vi "pressure system controller v18 numatics automated injection.vi"() -> ()   [LabVIEW 2015]
uses:
  <vilib>/DAQmx/write.llb/DAQmx Write (Digital 1D Bool 1Chan 1Samp).vi
  <vilib>/DAQmx/write.llb/DAQmx Write (Analog DBL 1Chan 1Samp).vi
  <vilib>/DAQmx/read.llb/DAQmx Read (Analog DBL 1Chan 1Samp).vi
  <vilib>/DAQmx/create/channels.llb/DAQmx Create Channel (AI-Voltage-Basic).vi
  <vilib>/DAQmx/configure/timing.llb/DAQmx Timing (Sample Clock).vi
  <vilib>/DAQmx/miscellaneous.llb/DAQmx Fill In Error Info.vi
  <vilib>/DAQmx/create/channels.llb/DAQmx Create Channel (AO-Voltage-Basic).vi
  <vilib>/DAQmx/create/channels.llb/DAQmx Create Channel (DO-Digital Output).vi
  <vilib>/express/express shared/transition.llb/Dynamic To Waveform Array.vi
  <vilib>/express/express signal manip/GetorSetDDTAttributes/Set DDT Attributes/SetT0.vi
  <vilib>/express/express shared/transition.llb/Waveform Array To Dynamic.vi
  <instrlib>/Keithley 24XX/Public/Data/Read (Single Point).vi
  <vilib>/express/express signal manip/GetorSetDDTAttributes/Set DDT Attributes/Set DDT Properties.xnode
  <vilib>/ptbypt/NI_PtbyPt.lvlib
  <instrlib>/Keithley 24XX/Keithley 24XX.lvlib
  <instrlib>/Agilent E4980/Agilent E4980.lvlib
panel:
  out "auto loop stop":bool
  in  "MUX1: LCR (+) 2":T1(radio)
  in  "Time Delay before current injection (s)":i32=5
  out "Inject Current":bool
  in  "Time Interval (sec)":i32=600
  in  "number of current inject":i32=5
  in  "Turn on (MAKE SURE TURN OFF)":bool=TRUE
  in  "MUX1: LCR (+)":T1(radio)
  in  "MUX2: LCR (-)":T1(radio)
  in  "MUX3: Keithley (+)":T1(radio)
  in  "MUX4: Keithley (-)":T1(radio)
  in  "Write to file":bool=TRUE caption="Enable"
  out "Pressure":dbl
  out "Impedance":dbl format="%^#_6e"
  out "Phase (deg)":dbl
  in  "Function (0: Cp-D)":u16(ring)=17 items=["Cp-D", "Cp-Q", "Cp-G", "Cp-Rp", "Cs-D", "Cs-Q", "Cs-Rs", "Lp-D", "Lp-Q", "Lp-G", "Lp-Rp", "Lp-Rdc", "Ls-D", "Ls-Q", "Ls-Rs", "Ls-Rdc", "R-X", "Z-thd", "Z-thr", "G-B", "Y-thd", "Y-thr", "Vdc-Idc"]
  in  "Signal Level (1.0 V)":dbl=1.0
  in  "Averaging Factor (1)":i32=1
  in  "Measurement Time (1: Medium)":u16(ring) items=["Short", "Medium", "Long"]
  in  "Signal Frequency":dbl=10000.0
  out "Resistance (Mohm)":dbl
  out "Current (uA)":sgl
  out "Voltage (V)":sgl
  in  "Loop sample rate (samples per second)":dbl=5.0
  in  "Current duration (s)":dbl=2.0
  out "Time Counter(s)":i32
  in  "Keithley Output (uA)":dbl=1.0
  in  "Compliance (V)":dbl=21.0
  out "Supply Current":dbl
  in  "Set Point Pressure (mmHg)":dbl min=0.0 max=500.0
  in  "stop":bool
  # "Keithley Settings"
  # "Pressure Setup"
  # "LCR Settings"
  # "1KHz for water"
  # "MAX: 75"
  # "10KHz for PBS"
  # "Automatic Control Panel"
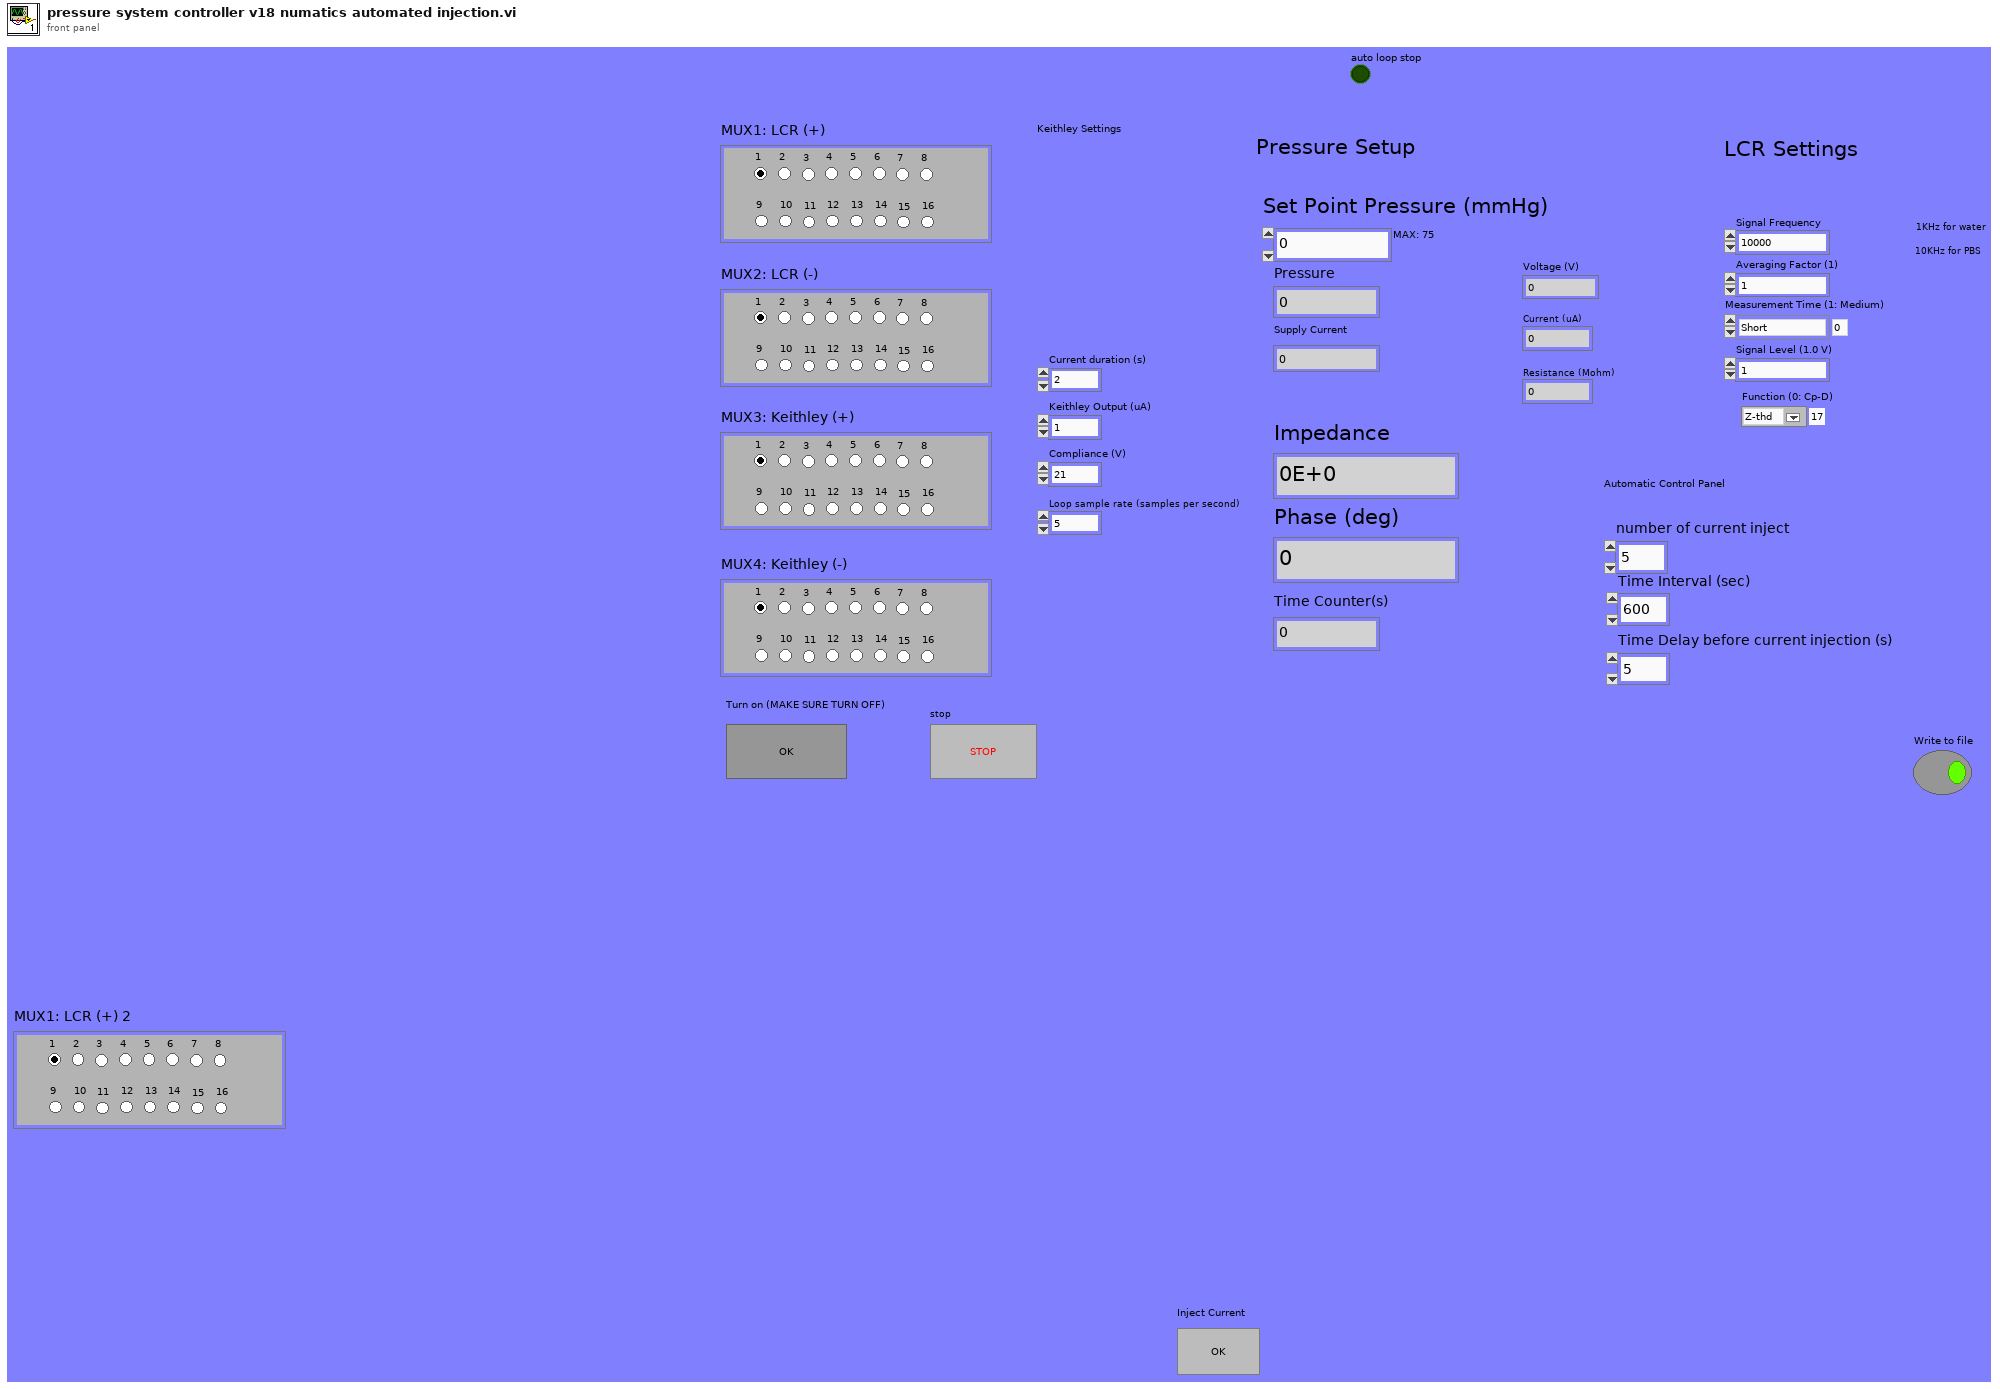
[diagram p1: front panel]
types:
  T1 = enum32{"1", "2", "3", "4", "5", "6", "7", "8", "9", "10", "11", "12", "13", "14", "15", "16"}
  T2 = cluster{"Primary Parameter":dbl, "Secondary Parameter":dbl}
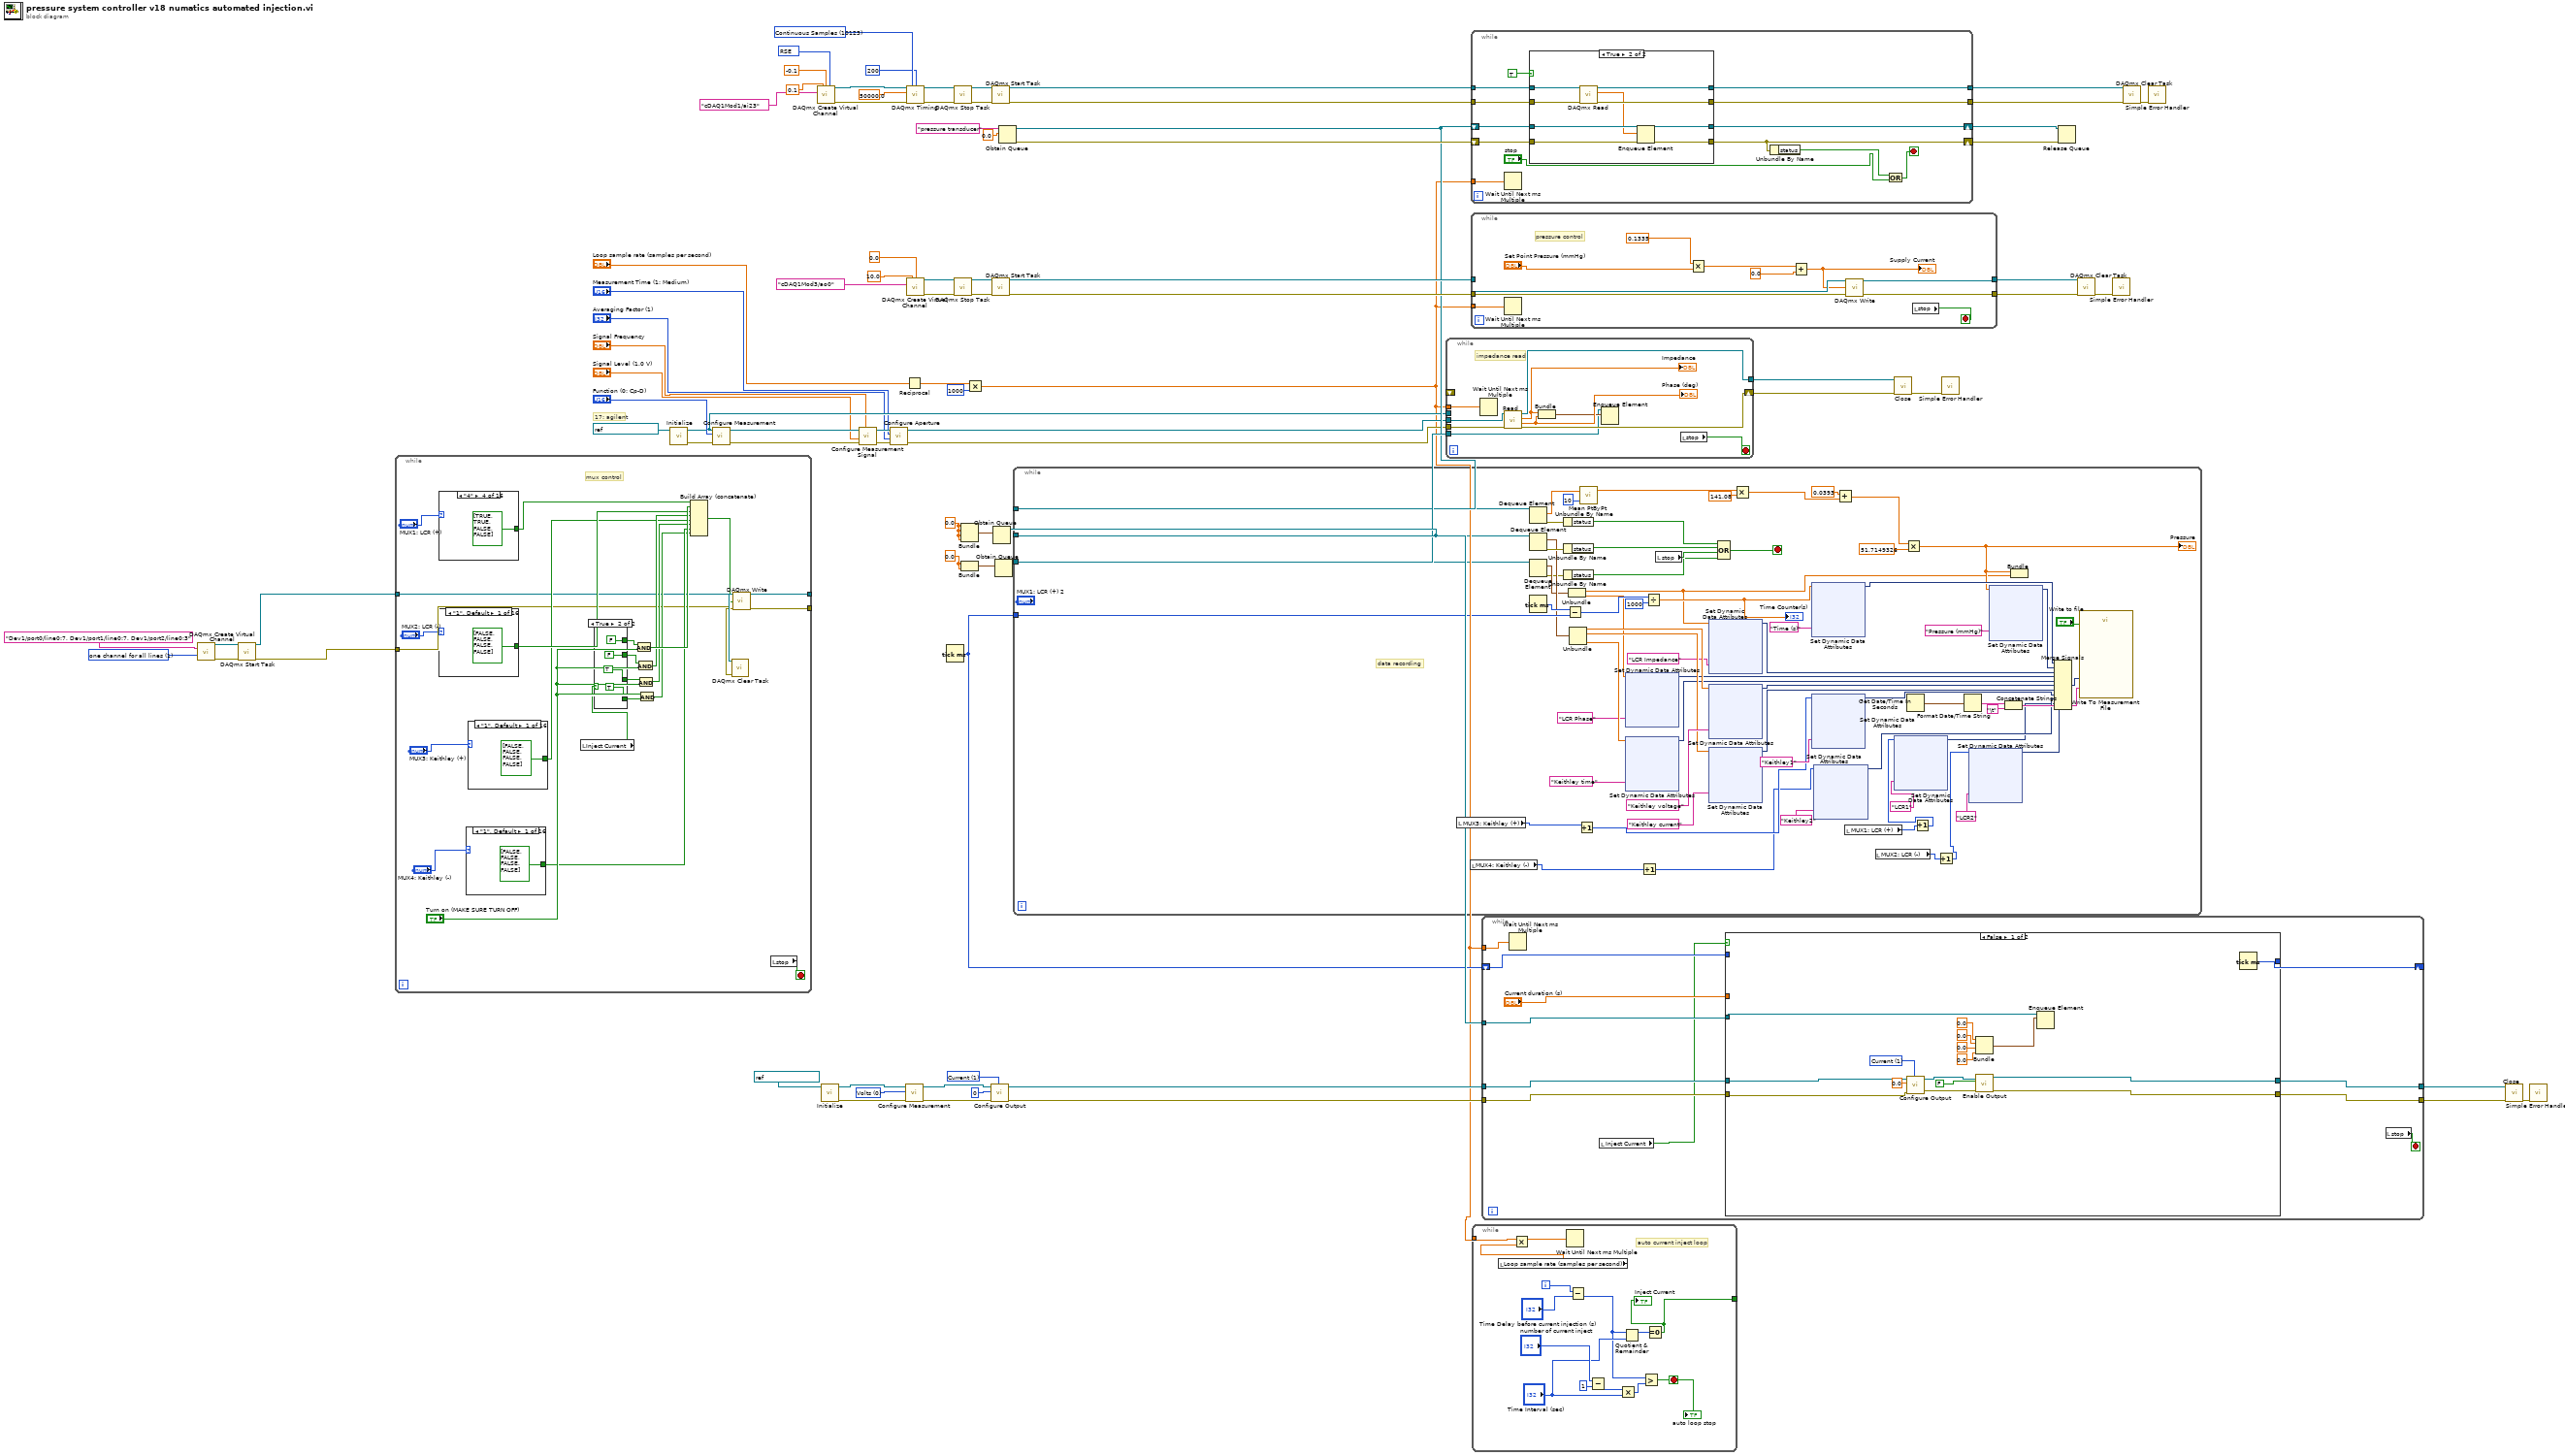
[diagram p0: block diagram]
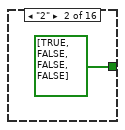
[diagram p2: hidden frame]
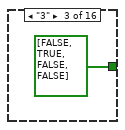
[diagram p3: hidden frame]
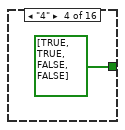
[diagram p4: hidden frame]
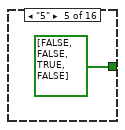
[diagram p5: hidden frame]
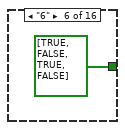
[diagram p6: hidden frame]
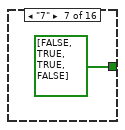
[diagram p7: hidden frame]
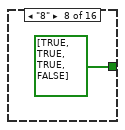
[diagram p8: hidden frame]
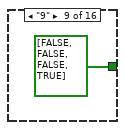
[diagram p9: hidden frame]
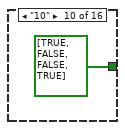
[diagram p10: hidden frame]
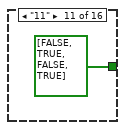
[diagram p11: hidden frame]
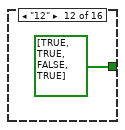
[diagram p12: hidden frame]
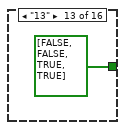
[diagram p13: hidden frame]
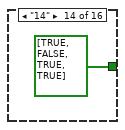
[diagram p14: hidden frame]
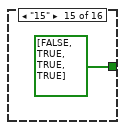
[diagram p15: hidden frame]
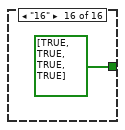
[diagram p16: hidden frame]
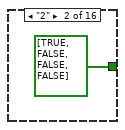
[diagram p17: hidden frame]
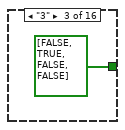
[diagram p18: hidden frame]
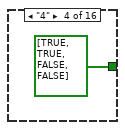
[diagram p19: hidden frame]
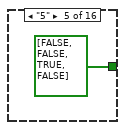
[diagram p20: hidden frame]
diagram:
  w9 = 1 items=["one channel for each line", "one channel for all lines"] ("line grouping")
  w48 = u16 1 items=["Voltage", "Current"] ("Source Mode  (0: Voltage)")
  w54 = u16 0 items=["Volts", "Current", "Resistance"] ("Keithley Measure")
  w34 = sgl 0.0 ("y")
  w42 = sgl 0.0 ("y")
  w82 = 10123 items=["Finite Samples"=10178, "Continuous Samples"=10123, "Hardware Timed Single Point"=12522] ("sample mode")
  w85 = 10083 items=["default"=-1, "RSE"=10083, "NRSE"=10078, "Differential"=10106, "Pseudodifferential"=12529] ("input terminal configuration")
  # "17: agilent"
  n1 = call-poly <vilib>:"DAQmx Create Virtual Channel.vi"("lines"=tag "Dev1/port0/line0:7, Dev1/port1/line0:7, Dev1/port2/line0:3", "line grouping"=w9) -> ("task out"=w7:refnum<k21>, "error out"=w8:errorcluster)  [unwired: 12 in]
  n2 = call <vilib>:"DAQmx Start Task.vi"("task/channels in"=w7, "error in"=w8) -> ("task out"=w5:refnum<k21>, "error out"=w3:errorcluster)  [unwired: 12 in]
  n3 = while {
    tunnel: w5 -> [w95]
    tunnel: [w94] -> w4
    tunnel: w3 -> [w93]
    tunnel: [w92] -> w2
    stop <- w108 stop-if-true
    # "mux control"
    n4 = case shown="\"4\"" "MUX1: LCR (+)" {
      tunnel: [bool[] [FALSE, FALSE, FALSE, FALSE] bool[] [TRUE, FALSE, FALSE, FALSE] bool[] [FALSE, TRUE, FALSE, FALSE] bool[] [TRUE, TRUE, FALSE, FALSE] bool[] [FALSE, FALSE, TRUE, FALSE] bool[] [TRUE, FALSE, TRUE, FALSE] bool[] [FALSE, TRUE, TRUE, FALSE] bool[] [TRUE, TRUE, TRUE, FALSE] bool[] [FALSE, FALSE, FALSE, TRUE] bool[] [TRUE, FALSE, FALSE, TRUE] bool[] [FALSE, TRUE, FALSE, TRUE] bool[] [TRUE, TRUE, FALSE, TRUE] bool[] [FALSE, FALSE, TRUE, TRUE] bool[] [TRUE, FALSE, TRUE, TRUE] bool[] [FALSE, TRUE, TRUE, TRUE] bool[] [TRUE, TRUE, TRUE, TRUE]] -> w103
      frame "1", Default {
      }
      frame "2" {
      }
      frame "3" {
      }
      frame "4" {
      }
      frame "5" {
      }
      frame "6" {
      }
      frame "7" {
      }
      frame "8" {
      }
      frame "9" {
      }
      frame "10" {
      }
      frame "11" {
      }
      frame "12" {
      }
      frame "13" {
      }
      frame "14" {
      }
      frame "15" {
      }
      frame "16" {
      }
    }
    n5 = case shown="\"1\", Default" "MUX2: LCR (-)" {
      tunnel: [bool[] [FALSE, FALSE, FALSE, FALSE] bool[] [TRUE, FALSE, FALSE, FALSE] bool[] [FALSE, TRUE, FALSE, FALSE] bool[] [TRUE, TRUE, FALSE, FALSE] bool[] [FALSE, FALSE, TRUE, FALSE] bool[] [TRUE, FALSE, TRUE, FALSE] bool[] [FALSE, TRUE, TRUE, FALSE] bool[] [TRUE, TRUE, TRUE, FALSE] bool[] [FALSE, FALSE, FALSE, TRUE] bool[] [TRUE, FALSE, FALSE, TRUE] bool[] [FALSE, TRUE, FALSE, TRUE] bool[] [TRUE, TRUE, FALSE, TRUE] bool[] [FALSE, FALSE, TRUE, TRUE] bool[] [TRUE, FALSE, TRUE, TRUE] bool[] [FALSE, TRUE, TRUE, TRUE] bool[] [TRUE, TRUE, TRUE, TRUE]] -> w101
      frame "1", Default {
      }
      frame "2" {
      }
      frame "3" {
      }
      frame "4" {
      }
      frame "5" {
      }
      frame "6" {
      }
      frame "7" {
      }
      frame "8" {
      }
      frame "9" {
      }
      frame "10" {
      }
      frame "11" {
      }
      frame "12" {
      }
      frame "13" {
      }
      frame "14" {
      }
      frame "15" {
      }
      frame "16" {
      }
    }
    n6 = case shown="\"1\", Default" "MUX4: Keithley (-)" {
      tunnel: [bool[] [FALSE, FALSE, FALSE, FALSE] bool[] [TRUE, FALSE, FALSE, FALSE] bool[] [FALSE, TRUE, FALSE, FALSE] bool[] [TRUE, TRUE, FALSE, FALSE] bool[] [FALSE, FALSE, TRUE, FALSE] bool[] [TRUE, FALSE, TRUE, FALSE] bool[] [FALSE, TRUE, TRUE, FALSE] bool[] [TRUE, TRUE, TRUE, FALSE] bool[] [FALSE, FALSE, FALSE, TRUE] bool[] [TRUE, FALSE, FALSE, TRUE] bool[] [FALSE, TRUE, FALSE, TRUE] bool[] [TRUE, TRUE, FALSE, TRUE] bool[] [FALSE, FALSE, TRUE, TRUE] bool[] [TRUE, FALSE, TRUE, TRUE] bool[] [FALSE, TRUE, TRUE, TRUE] bool[] [TRUE, TRUE, TRUE, TRUE]] -> w97
      frame "1", Default {
      }
      frame "2" {
      }
      frame "3" {
      }
      frame "4" {
      }
      frame "5" {
      }
      frame "6" {
      }
      frame "7" {
      }
      frame "8" {
      }
      frame "9" {
      }
      frame "10" {
      }
      frame "11" {
      }
      frame "12" {
      }
      frame "13" {
      }
      frame "14" {
      }
      frame "15" {
      }
      frame "16" {
      }
    }
    n7 = case shown="\"1\", Default" "MUX3: Keithley (+)" {
      tunnel: [bool[] [FALSE, FALSE, FALSE, FALSE] bool[] [TRUE, FALSE, FALSE, FALSE] bool[] [FALSE, TRUE, FALSE, FALSE] bool[] [TRUE, TRUE, FALSE, FALSE] bool[] [FALSE, FALSE, TRUE, FALSE] bool[] [TRUE, FALSE, TRUE, FALSE] bool[] [FALSE, TRUE, TRUE, FALSE] bool[] [TRUE, TRUE, TRUE, FALSE] bool[] [FALSE, FALSE, FALSE, TRUE] bool[] [TRUE, FALSE, FALSE, TRUE] bool[] [FALSE, TRUE, FALSE, TRUE] bool[] [TRUE, TRUE, FALSE, TRUE] bool[] [FALSE, FALSE, TRUE, TRUE] bool[] [TRUE, FALSE, TRUE, TRUE] bool[] [FALSE, TRUE, TRUE, TRUE] bool[] [TRUE, TRUE, TRUE, TRUE]] -> w99
      frame "1", Default {
      }
      frame "2" {
      }
      frame "3" {
      }
      frame "4" {
      }
      frame "5" {
      }
      frame "6" {
      }
      frame "7" {
      }
      frame "8" {
      }
      frame "9" {
      }
      frame "10" {
      }
      frame "11" {
      }
      frame "12" {
      }
      frame "13" {
      }
      frame "14" {
      }
      frame "15" {
      }
      frame "16" {
      }
    }
    n8 = local read "Inject Current"() -> (w90:bool)
    n9 = case shown="True" w90 {
      tunnel: [TRUE FALSE] -> w107
      tunnel: [TRUE FALSE] -> w106
      tunnel: [FALSE TRUE] -> w105
      tunnel: [FALSE TRUE] -> w104
      frame False {
      }
      frame True {
      }
    }
    n10 = And(x=w107, y="Turn on (MAKE SURE TURN OFF)") -> (x .and. y?=w102:bool)
    n11 = And(x=w106, y="Turn on (MAKE SURE TURN OFF)") -> (x .and. y?=w100:bool)
    n12 = And(x=w105, y="Turn on (MAKE SURE TURN OFF)") -> (x .and. y?=w98:bool)
    n13 = And(x="Turn on (MAKE SURE TURN OFF)", y=w104) -> (x .and. y?=w96:bool)
    n14 = Build Array (concatenate)(w103, w102, w101, w100, w99, w98, w97, w96) -> (w91:bool[])
    n15 = call-poly <vilib>:"DAQmx Write.vi"("task/channels in"=w95, "data"=w91, "error in"=w93) -> ("task out"=w94:refnum<k21>, "error out"=w92:errorcluster)  [unwired: 10 in, 1 out]
    n16 = local read "stop"() -> (w108:bool)
  }
  n17 = call <instrlib>:"Initialize.vi"("VISA resource name"=refnum<visa-resource-name> "GPIB0::16::INSTR") -> ("error out"=w25:errorcluster, "VISA resource name out"=w24:refnum<visa-resource-name>)  [unwired: 9 in]
  n18 = call <instrlib>:"Configure Measurement.vi"("error in (no error)"=w25, "Function (0: Cp-D)"="Function (0: Cp-D)", "VISA resource name"=w24) -> ("error out"=w23:errorcluster, "VISA resource name out"=w22:refnum<visa-resource-name>)  [unwired: 7 in]
  n19 = call <vilib>:"DAQmx Clear Task.vi"("task in"=w4, "error in"=w2) -> ()  [unwired: 13 in, 1 out]
  n20 = call-poly <vilib>:"DAQmx Create Virtual Channel.vi"("maximum value"=0.1, "minimum value"=-0.1, "input terminal configuration"=w85, "physical channels"=tag "cDAQ1Mod1/ai23") -> ("task out"=w79:refnum<k21>, "error out"=w78:errorcluster)  [unwired: 10 in]
  n21 = call <instrlib>:"Initialize.vi"("VISA resource name"=refnum<visa-resource-name> "GPIB0::24::INSTR") -> ("error out"=w52:errorcluster, "VISA resource name out"=w53:refnum<visa-resource-name>)  [unwired: 9 in]
  n22 = call <instrlib>:"Configure Measurement Signal.vi"("Signal Frequency (1000 Hz)"="Signal Frequency", "error in (no error)"=w23, "Signal Level (1.0 V)"="Signal Level (1.0 V)", "VISA resource name"=w22) -> ("error out"=w19:errorcluster, "VISA resource name out"=w18:refnum<visa-resource-name>)  [unwired: 6 in]
  n23 = call <instrlib>:"Configure Aperture.vi"("error in (no error)"=w19, "Averaging Factor (1)"="Averaging Factor (1)", "Measurement Time (1: Medium)"="Measurement Time (1: Medium)", "VISA resource name"=w18) -> ("error out"=w15:errorcluster, "VISA resource name out"=w14:refnum<visa-resource-name>)  [unwired: 6 in]
  n24 = call <instrlib>:"Configure Measurement.vi"("error in (no error)"=w52, "Function (0: Volts)"=w54, "VISA resource name"=w53) -> ("error out"=w50:errorcluster, "VISA resource name out"=w51:refnum<visa-resource-name>)  [unwired: 7 in]
  n25 = Reciprocal(x="Loop sample rate (samples per second)") -> (1/x=w39:dbl)
  n26 = call-poly <vilib>:"DAQmx Timing.vi"("task/channels in"=w79, "sample mode"=w82, "samples per channel"=200, "rate"=50000.0, "error in"=w78) -> ("task out"=w77:refnum<k21>, "error out"=w76:errorcluster)  [unwired: 9 in]
  n27 = call-poly <vilib>:"DAQmx Create Virtual Channel.vi"("maximum value"=10.0, "minimum value"=0.0, "physical channels"=tag "cDAQ1Mod3/ao0") -> ("task out"=w60:refnum<k21>, "error out"=w59:errorcluster)  [unwired: 11 in]
  n28 = Tick Count (ms)() -> (millisecond timer value=w12:u32)
  n29 = call <vilib>:"DAQmx Stop Task.vi"("task/channels in"=w77, "error in"=w76) -> ("task out"=w75:refnum<k21>, "error out"=w74:errorcluster)  [unwired: 12 in]
  n30 = call <vilib>:"DAQmx Stop Task.vi"("task/channels in"=w60, "error in"=w59) -> ("task out"=w62:refnum<k21>, "error out"=w61:errorcluster)  [unwired: 12 in]
  n31 = Bundle("y"=w42, "y"=w42, "y"=w42, "y"=w42) -> (w41:cluster{"y":sgl, "y":sgl, "y":sgl, "y":sgl})  [unwired: 1 in]
  n32 = Bundle("y"=w34, "y"=w34) -> (w33:cluster{"y":sgl, "y":sgl})  [unwired: 1 in]
  n33 = Multiply(x=w39, y=1000) -> (x*y=w1:dbl)
  n34 = call <instrlib>:"Configure Output.vi"("Source Mode  (0: Voltage)"=w48, "error in (no error)"=w50, "Output Level (0)"=0, "VISA resource name"=w51) -> ("error out"=w46:errorcluster, "VISA resource name out"=w47:refnum<visa-resource-name>)  [unwired: 6 in]
  n35 = call <vilib>:"DAQmx Start Task.vi"("task/channels in"=w75, "error in"=w74) -> ("task out"=w69:refnum<k21>, "error out"=w68:errorcluster)  [unwired: 12 in]
  n36 = call <vilib>:"DAQmx Start Task.vi"("task/channels in"=w62, "error in"=w61) -> ("task out"=w58:refnum<k21>, "error out"=w57:errorcluster)  [unwired: 12 in]
  n37 = Obtain Queue(element data type=w41) -> (queue out=w45:refnum<queue>)  [unwired: 4 in, 2 out]
  n38 = Obtain Queue(element data type=w33) -> (queue out=w32:refnum<queue>)  [unwired: 4 in, 2 out]
  n39 = Obtain Queue(name (unnamed)="pressure transducer", element data type=sgl 0.0 ("kvoltage")) -> (queue out=w27:refnum<queue>, error out=w73:errorcluster)  [unwired: 3 in, 1 out]
  n40 = while {
    tunnel: w27 -> [w248]
    tunnel: w12 -> [w236]
    tunnel: w45 -> [w232]
    tunnel: w32 -> [w217]
    stop <- w228 stop-if-true
    # "data recording"
    n41 = local read "MUX3: Keithley (+)"() -> (w189:T1)
    n42 = local read "MUX4: Keithley (-)"() -> (w186:T1)
    n43 = Dequeue Element(queue=w248) -> (element=w210:sgl, error out=w249:errorcluster)  [unwired: 2 in, 2 out]
    n44 = Dequeue Element(queue=w232) -> (element=w227:cluster{"y":sgl, "y":sgl, "y":sgl, "y":sgl}, error out=w231:errorcluster)  [unwired: 2 in, 2 out]
    n45 = Dequeue Element(queue=w217) -> (element=w216:cluster{"y":sgl, "y":sgl}, error out=w212:errorcluster)  [unwired: 2 in, 2 out]
    n46 = Tick Count (ms)() -> (millisecond timer value=w239:u32)
    n47 = Unbundle By Name(w249) -> ("status"=w230:bool)
    n48 = Unbundle By Name(w231) -> ("status"=w229:bool)
    n49 = Unbundle By Name(w212) -> ("status"=w211:bool)
    n50 = Subtract(x=w239, y=w236) -> (x-y=w237:u32)
    n51 = Unbundle(w216) -> ("y"=w213:sgl, "y"=w215:sgl)
    n52 = Unbundle(w227) -> ("y"=w222:sgl, "y"=w221:sgl, "y"=w223:sgl)  [unwired: 1 out]
    n53 = Increment(x=w189) -> (x+1=w188:T1)
    n54 = call <vilib>:"Mean PtByPt.vi"("x"=w210, "sample length"=10) -> ("mean"=w203:dbl)  [unwired: 2 in, 1 out]
    n55 = xnode "Set Dynamic Data Attributes"("Signal Name"="LCR Phase", "Signals In"=w215) -> ("Signals Out"=w207:dynamicdata)  [unwired: 2 in, 1 out]
    n56 = xnode "Set Dynamic Data Attributes"("Signal Name"="Keithley time", "Signals In"=w223) -> ("Signals Out"=w206:dynamicdata)  [unwired: 2 in, 1 out]
    n57 = Increment(x=w186) -> (x+1=w187:T1)
    n58 = Divide(x=w237, y=1000) -> (x/y=w234:dbl)
    "Time Counter(s)" <- w234
    n59 = local read "stop"() -> (w220:bool)
    n60 = xnode "Set Dynamic Data Attributes"("Signal Name"="LCR Impedance", "Signals In"=w213) -> ("Signals Out"=w208:dynamicdata)  [unwired: 2 in, 1 out]
    n61 = xnode "Set Dynamic Data Attributes"("Signal Name"="Keithley voltage", "Signals In"=w222) -> ("Signals Out"=w205:dynamicdata)  [unwired: 2 in, 1 out]
    n62 = xnode "Set Dynamic Data Attributes"("Signal Name"="Keithley current", "Signals In"=w221) -> ("Signals Out"=w204:dynamicdata)  [unwired: 2 in, 1 out]
    n63 = Compound Arithmetic op=OR(w230, w229, w220, w211) -> (w228:bool)
    n64 = Multiply(x=w203, y=141.08) -> (x*y=w201:dbl)
    n65 = xnode "Set Dynamic Data Attributes"("Signal Name"="Time (s)", "Signals In"=w234) -> ("Signals Out"=w233:dynamicdata)  [unwired: 2 in, 1 out]
    n66 = xnode "Set Dynamic Data Attributes"("Signal Name"="Keithley1", "Signals In"=w188) -> ("Signals Out"=w197:dynamicdata)  [unwired: 2 in, 1 out]
    n67 = xnode "Set Dynamic Data Attributes"("Signal Name"="Keithley2", "Signals In"=w187) -> ("Signals Out"=w196:dynamicdata)  [unwired: 2 in, 1 out]
    n68 = Add(x=0.0393, y=w201) -> (x+y=w199:dbl)
    n69 = local read "MUX1: LCR (+)"() -> (w185:T1)
    n70 = local read "MUX2: LCR (-)"() -> (w183:T1)
    n71 = Multiply(x=w199, y=51.7149326) -> (x*y=w214:dbl)
    "Pressure" <- w214
    n72 = Get Date/Time In Seconds() -> (seconds since 1Jan1904=w243:timestamp)
    n73 = Increment(x=w185) -> (x+1=w184:T1)
    n74 = xnode "Set Dynamic Data Attributes"("Signal Name"="LCR1", "Signals In"=w184) -> ("Signals Out"=w195:dynamicdata)  [unwired: 2 in, 1 out]
    n75 = Increment(x=w183) -> (x+1=w182:T1)
    n76 = Format Date/Time String(seconds (now)=w243) -> (date/time string=w244:string)  [unwired: 2 in]
    n77 = xnode "Set Dynamic Data Attributes"("Signal Name"="LCR2", "Signals In"=w182) -> ("Signals Out"=w194:dynamicdata)  [unwired: 2 in, 1 out]
    n78 = xnode "Set Dynamic Data Attributes"("Signal Name"="Pressure (mmHg)", "Signals In"=w214) -> ("Signals Out"=w241:dynamicdata)  [unwired: 2 in, 1 out]
    n79 = Concatenate Strings(w244, "\t") -> (w242:string)
    n80 = Bundle(w214, "y"=w213) -> ()  [unwired: 1 in, 1 out]
    n81 = Merge Signals(w233, w241, w208, w207, w206, w205, w204, w197, w196, w195, w194) -> (w240:dynamicdata)
    n82 = call "Write To Measurement File"("Signals"=w240, "Enable"="Write to file", "Comment"=w242) -> ()  [unwired: 14 in, 3 out]
  }
  n83 = while {
    shift-right: [w413] -> w36
    shift-left: _ -> [_]
    tunnel: w24 -> [_]
    tunnel: [w412] -> w35
    tunnel: w1 -> [w411]
    tunnel: w32 -> [w407]
    tunnel: w15 -> [w405]
    tunnel: w14 -> [w404]
    stop <- w406 stop-if-true
    # "impedance read"
    n84 = Wait Until Next ms Multiple(millisecond multiple=w411) -> ()  [unwired: 1 out]
    n85 = call <instrlib>:"Read.vi"("error in (no error)"=w405, "VISA resource name"=w404) -> ("error out"=w413:errorcluster, "Secondary Parameter"=w410:dbl, "Primary Parameter"=w409:dbl, "VISA resource name out"=w412:refnum<visa-resource-name>)  [unwired: 6 in]
    "Phase (deg)" <- w410
    "Impedance" <- w409
    n86 = Bundle("Primary Parameter"=w409, "Secondary Parameter"=w410) -> (w408:T2)  [unwired: 1 in]
    n87 = Enqueue Element(queue=w407, element=w408) -> ()  [unwired: 2 in, 3 out]
    n88 = local read "stop"() -> (w406:bool)
  }
  n89 = while {
    shift-right: [w423] -> w71
    shift-left: w73 -> [w425]
    tunnel: w69 -> [w422]
    tunnel: w68 -> [w421]
    tunnel: [w420] -> w67
    tunnel: [w419] -> w66
    shift-right: [w424] -> w72
    shift-left: w27 -> [w426]
    tunnel: w1 -> [w418]
    stop <- w414 stop-if-true
    n90 = Wait Until Next ms Multiple(millisecond multiple=w418) -> ()  [unwired: 1 out]
    n91 = case shown="True" TRUE {
      tunnel: w426 -> [w430 w439]
      tunnel: w425 -> [w429 w438]
      tunnel: [w430 w437] -> w424
      tunnel: [w429 w436] -> w423
      tunnel: w422 -> [w428 w435]
      tunnel: w421 -> [w427 w434]
      tunnel: [w428 w433] -> w420
      tunnel: [w427 w432] -> w419
      frame False {
      }
      frame True {
        n92 = call-poly <vilib>:"DAQmx Read.vi"("task/channels in"=w435, "error in"=w434) -> ("task out"=w433:refnum<k21>, "data"=w431:dbl, "error out"=w432:errorcluster)  [unwired: 11 in]
        n93 = Enqueue Element(queue=w439, element=w431, error in (no error)=w438) -> (queue out=w437:refnum<queue>, error out=w436:errorcluster)  [unwired: 1 in, 1 out]
      }
    }
    n94 = Unbundle By Name(w423) -> ("status"=w416:bool)
    n95 = Compound Arithmetic op=OR(w416, "stop") -> (w414:bool)
  }
  n96 = while {
    tunnel: w58 -> [w450]
    tunnel: w57 -> [w449]
    tunnel: [w448] -> w56
    tunnel: [w447] -> w55
    tunnel: w1 -> [w445]
    stop <- w446 stop-if-true
    # "pressure control"
    n97 = Wait Until Next ms Multiple(millisecond multiple=w445) -> ()  [unwired: 1 out]
    n98 = Multiply(x=0.1335, y="Set Point Pressure (mmHg)") -> (x*y=w443:dbl)
    n99 = Add(x=w443, y=0.0) -> (x+y=w441:dbl)
    "Supply Current" <- w441
    n100 = call-poly <vilib>:"DAQmx Write.vi"("task/channels in"=w450, "data"=w441, "error in"=w449) -> ("task out"=w448:refnum<k21>, "error out"=w447:errorcluster)  [unwired: 10 in, 1 out]
    n101 = local read "stop"() -> (w446:bool)
  }
  n102 = while {
    tunnel: [w457] -> _
    tunnel: w1 -> [w458]
    i -> [w452]
    stop <- w464 stop-if-true
    # "auto current inject loop"
    n103 = local read "Loop sample rate (samples per second)"() -> (w455:dbl)
    n104 = Multiply(x=w458, y=w455) -> (x*y=w456:dbl)
    n105 = Wait Until Next ms Multiple(millisecond multiple=w456) -> ()  [unwired: 1 out]
    n106 = Subtract(x=w452, y="Time Delay before current injection (s)") -> (x-y=w453:i32)
    n107 = Subtract(x="number of current inject", y=1 ("x")) -> (x-y=w460:i32)
    n108 = Multiply(x=w460, y="Time Interval (sec)") -> (x*y=w463:i32)
    n109 = Quotient & Remainder(x=w453, y="Time Interval (sec)") -> (x-y*floor(x/y)=w461:i32)  [unwired: 1 out]
    n110 = Greater?(x=w453, y=w463) -> (0:w464:bool)
    "auto loop stop" <- w464
    n111 = Equal To 0?(x=w461) -> (x = 0?=w457:bool)
    "Inject Current" <- w457
  }
  n112 = while {
    tunnel: w47 -> [w475]
    tunnel: w46 -> [w474]
    tunnel: w45 -> [w472]
    tunnel: [w467] -> w44
    tunnel: [w466] -> w43
    shift-right: [w470] -> _
    shift-left: w12 -> [w469]
    tunnel: w1 -> [w468]
    stop <- w473 stop-if-true
    n113 = Wait Until Next ms Multiple(millisecond multiple=w468) -> ()  [unwired: 1 out]
    n114 = local read "Inject Current"() -> (w465:bool)
    n115 = case shown="False" w465 {
      tunnel: w475 -> [w481 w522]
      tunnel: w474 -> [w480 w521]
      tunnel: w472 -> [w489 w514]
      tunnel: "Current duration (s)" -> [_ w512]
      tunnel: [w491 w507] -> w467
      tunnel: [w490 w506] -> w466
      tunnel: [w483 w504] -> w470
      tunnel: w469 -> [_ w504]
      frame False {
        w476 = u16 1 items=["Voltage", "Current"] ("Source Mode  (0: Voltage)")
        n116 = call <instrlib>:"Configure Output.vi"("Source Mode  (0: Voltage)"=w476, "error in (no error)"=w480, "Output Level (0)"=0.0, "VISA resource name"=w481) -> ("error out"=w478:errorcluster, "VISA resource name out"=w479:refnum<visa-resource-name>)  [unwired: 6 in]
        n117 = Bundle("y"=sgl 0.0, "y"=sgl 0.0, "y"=sgl 0.0, "y"=sgl 0.0) -> (w488:cluster{"y":sgl, "y":sgl, "y":sgl, "y":sgl})  [unwired: 1 in]
        n118 = call <instrlib>:"Enable Output.vi"("error in (no error)"=w478, "Enable Output (T: Enable)"=FALSE, "VISA resource name"=w479) -> ("error out"=w490:errorcluster, "VISA resource name out"=w491:refnum<visa-resource-name>)  [unwired: 7 in]
        n119 = Enqueue Element(queue=w489, element=w488) -> ()  [unwired: 2 in, 3 out]
        n120 = Tick Count (ms)() -> (millisecond timer value=w483:u32)
      }
      frame True {
        w497 = u16 1 items=["Voltage", "Current"] ("Source Mode  (0: Voltage)")
        n121 = Tick Count (ms)() -> (millisecond timer value=w505:u32)
        n122 = Subtract(x=w505, y=w504) -> (x-y=w500:u32)
        n123 = call <instrlib>:"Enable Output.vi"("error in (no error)"=w521, "Enable Output (T: Enable)"=TRUE, "VISA resource name"=w522) -> ("error out"=w498:errorcluster, "VISA resource name out"=w499:refnum<visa-resource-name>)  [unwired: 7 in]
        n124 = Divide(x=w500, y=1000) -> (x/y=w510:dbl)
        n125 = Multiply(x="Keithley Output (uA)", y=1e-06) -> (x*y=w501:dbl)
        n126 = Greater Or Equal?(x=w510, y=w512) -> (x >= y?=w511:bool)
        n127 = Not(x=w511) -> (.not. x?=w492:bool)
        n128 = call <instrlib>:"Configure Output.vi"("Source Mode  (0: Voltage)"=w497, "error in (no error)"=w498, "Compliance  Level (0.1)"="Compliance (V)", "Output Level (0)"=w501, "VISA resource name"=w499) -> ("error out"=w494:errorcluster, "VISA resource name out"=w495:refnum<visa-resource-name>)  [unwired: 5 in]
        n129 = call-poly <instrlib>:"Read.vi"("VISA resource name"=w495, "error in (no error)"=w494) -> ("Voltage"=w509:sgl, "VISA resource name out"=w507:refnum<visa-resource-name>, "Current"=w520:sgl, "Resistance"=w518:sgl, "error out"=w506:errorcluster)  [unwired: 7 in, 2 out]
        "Voltage (V)" <- w509
        n130 = local write "Inject Current"(w492) -> ()
        n131 = Multiply(x=w518, y=1e-06) -> (x*y=w516:dbl)
        "Resistance (Mohm)" <- w516
        n132 = Multiply(x=w520, y=sgl 1000000.0) -> (x*y=w508:sgl)
        "Current (uA)" <- w508
        n133 = Bundle("Voltage"=w509, w508, w516, w510) -> (w515:cluster{"Voltage":sgl, sgl, dbl, dbl})  [unwired: 1 in]
        n134 = Enqueue Element(queue=w514, element=w515) -> ()  [unwired: 2 in, 3 out]
      }
    }
    n135 = local read "stop"() -> (w473:bool)
  }
  n136 = call <instrlib>:"Close.vi"("error in (no error)"=w36, "VISA resource name"=w35) -> ("error out"=w30:errorcluster)  [unwired: 9 in]
  n137 = call <vilib>:"Simple Error Handler.vi"("error in (no error)"=w30) -> ()  [unwired: 4 in, 5 out]
  n138 = Release Queue(queue=w72, error in (no error)=w71) -> ()  [unwired: 1 in, 3 out]
  n139 = call <vilib>:"DAQmx Clear Task.vi"("task in"=w56, "error in"=w55) -> ("error out"=w28:errorcluster)  [unwired: 13 in]
  n140 = call <vilib>:"Simple Error Handler.vi"("error in (no error)"=w28) -> ()  [unwired: 4 in, 5 out]
  n141 = call <vilib>:"DAQmx Clear Task.vi"("task in"=w67, "error in"=w66) -> ("error out"=w29:errorcluster)  [unwired: 13 in]
  n142 = call <vilib>:"Simple Error Handler.vi"("error in (no error)"=w29) -> ()  [unwired: 4 in, 5 out]
  n143 = call <instrlib>:"Close.vi"("error in (no error)"=w43, "VISA resource name"=w44) -> ("error out"=w31:errorcluster)  [unwired: 9 in]
  n144 = call <vilib>:"Simple Error Handler.vi"("error in (no error)"=w31) -> ()  [unwired: 4 in, 5 out]
